vi "Get Screen Size.vi"() -> (2 "height":i16, 3 "width":i16)   [LabVIEW 2023, in "Winsys.lvlib"]
doc: "Gets the size of the screen in pixels."
uses:
  Winsys.lvlib
  user32.dll
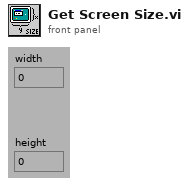
[diagram p1: front panel]
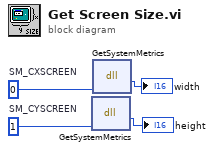
[diagram p0: block diagram]
diagram:
  w3 = 1  # SM_CYSCREEN
  w4 = 0  # SM_CXSCREEN
  n1 = dll-call lib="USER32.DLL" fn="GetSystemMetrics"("parameter"=w3) -> ("screenHeight"=→"height":i32)  [unwired: 4 in, 2 out]
  n2 = dll-call lib="USER32.DLL" fn="GetSystemMetrics"("parameter"=w4) -> ("screenWidth"=→"width":i32)  [unwired: 4 in, 2 out]
